vi "Get Hierarchy Item List.vi"(8 "error in (no error)":errorcluster, 11 "Item Reference in":T1 format="%.0x") -> (0 "error out":errorcluster, 1 "Item References out":T1[](array[typedef]) format="%.0x", 2 "Item Names out":string[](array[string]), 3 "Item Reference out":T1 format="%.0x")   [LabVIEW 2013]
uses:
  Item/Ctls/Item Reference.ctl
  Section/Section.lvclass
  Item/Item.lvclass
panel:
  # "获取当前节点下所包含的所有节点名称及引用"
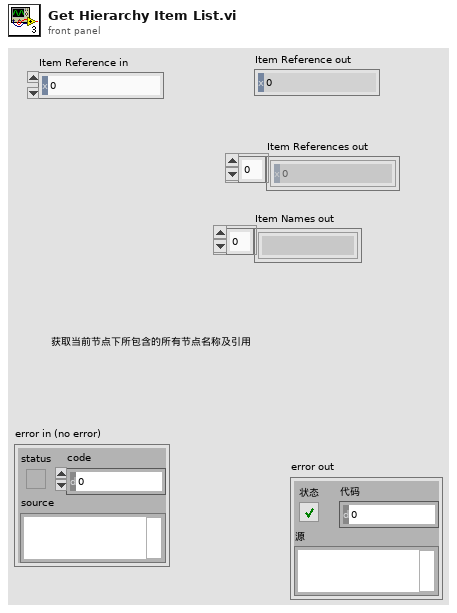
[diagram p1: front panel]
types:
  T1 = typedef "Hierarchy Framework.lvlib/Item.lvclass/Item Reference.ctl" = u64
  T2 = typedef "Hierarchy Framework.lvlib/Item.lvclass/Item Info.ctl" = cluster{"Name":string, "TagGUID":string, "TypeGUID":string, "Enable":bool}
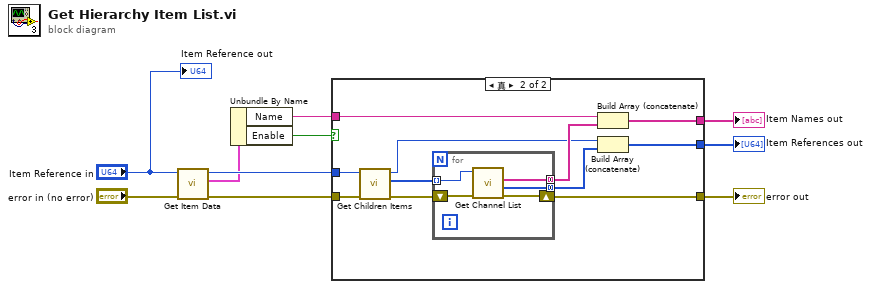
[diagram p0: block diagram]
diagram:
  n1 = call "Get Item Data.vi"("error in (no error)"="error in (no error)", "Item Reference in"="Item Reference in") -> ("error out"=w10:errorcluster, "Item Info"=w7:T2, "Item Reference out"=w8:T1)  [unwired: 6 in, 1 out]
  n2 = Unbundle By Name(w7) -> ("Name"=w4:string, "Enable"=w5:bool)
  n3 = case shown="真" w5 {
    tunnel: w10 -> [w11 w22]
    tunnel: w8 -> [_ w21]
    tunnel: [w11 w20] -> w6
    tunnel: w4 -> [_ w17]
    tunnel: [_ w13] -> w2
    tunnel: [_ w12] -> w1
    frame False {
    }
    frame True {
      n4 = call "Get Children Items.vi"("error in (no error)"=w22, "Section Reference in"=w21) -> ("error out"=w19:errorcluster, "Children Item References"=w18:u64[], "Section Reference out"=w14:u64)  [unwired: 5 in, 2 out]
      n5 = for {
        tunnel: w18 -> [w25] mode=indexing
        shift-right: [w26] -> w20
        shift-left: w19 -> [w27]
        tunnel: [w24] -> w16 mode=concatenating
        tunnel: [w23] -> w15 mode=concatenating
        n6 = call "Get Channel List.vi"("error in (no error)"=w27, "Item Reference in"=w25) -> ("error out"=w26:errorcluster, "Item References out"=w23:T1[], "Item Names out"=w24:string[])  [unwired: 6 in, 1 out]
      }
      n7 = Build Array (concatenate)(w17, w16) -> (w13:string[])
      n8 = Build Array (concatenate)(w14, w15) -> (w12:T1[])
    }
  }
  "Item References out" <- w1
  "Item Names out" <- w2
  "error out" <- w6
  "Item Reference out" <- "Item Reference in"
